vi "Set Error Codes File Properties.vi"(8 "error in (no error)":errorcluster, 10 "properties":T1, 11 "error list <owner> in":variant) -> (0 "error out":errorcluster, 3 "error list <owner> out":variant)   [LabVIEW 2017]
uses:
  Error Code File Properties.ctl
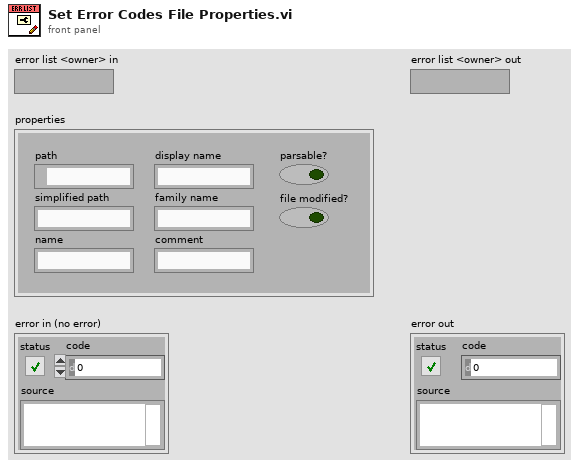
[diagram p1: front panel]
types:
  T1 = typedef "Error Code File Properties.ctl" = cluster{"path":path, "simplified path":string, "name":string, "display name":string, "family name":string, "comment":string, "parsable?":bool, "file modified?":bool}
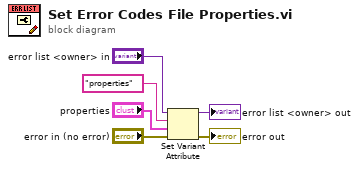
[diagram p0: block diagram]
diagram:
  n1 = Set Variant Attribute(Variant="error list <owner> in", name="properties", value="properties", error in="error in (no error)") -> (Variant out=→"error list <owner> out":variant, error out=→"error out":errorcluster)  [unwired: 1 out]
